vi "Auto Intake Mode.vi"   [LabVIEW 2017]
uses:
  Robot Global Data.vi
types:
  T1 = typedef "Intake Command Cluster.ctl" = cluster{"Intake Mode":T2, "Intake States":T3}
  T2 = typedef "Intake Mode.ctl" = enum16{"Auto", "Manual"}
  T3 = typedef "Intake States.ctl" = enum16{"Idle", "Intake", "Outtake"}
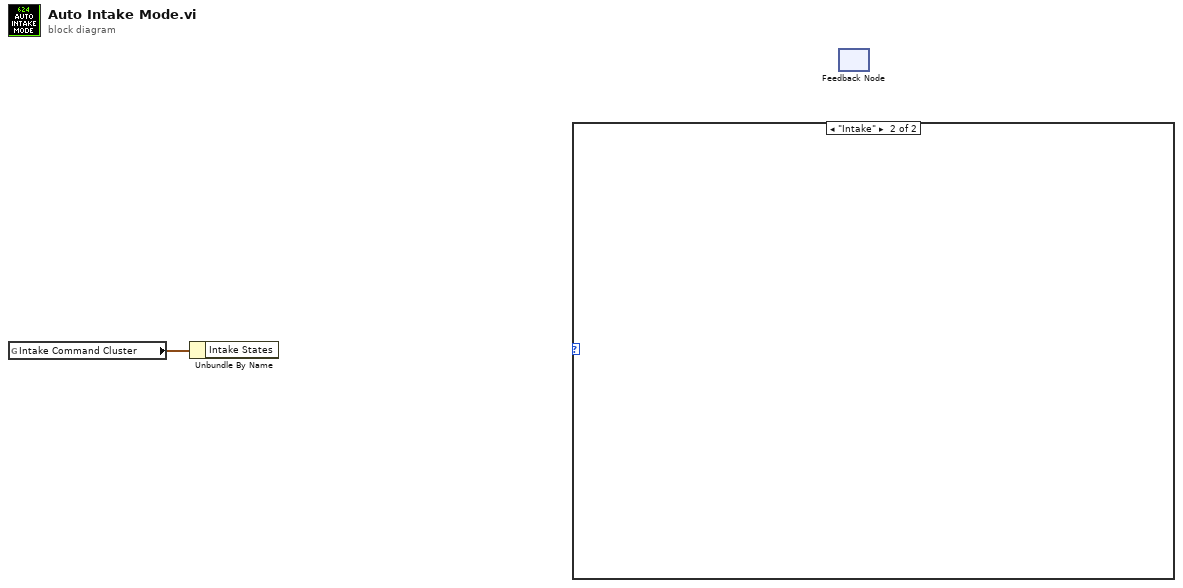
[diagram p0: block diagram]
diagram:
  n1 = global read "Robot Global Data.vi" "Intake Command Cluster"() -> (w1:T1)
  n2 = Unbundle By Name(w1) -> ()  [unwired: 1 out]
  n3 = case shown="\"Intake\"" {
    selector: _ -> [_ _]
    frame "Idle", Default {
    }
    frame "Intake" {
    }
  }
  n4 = feedback-in #1() -> ()  [unwired: 1 out]
  n5 = feedback #1() -> ()  [unwired: 2 in]
